vi "prroducer and consumer design patterrn.vi"() -> ()   [LabVIEW 2022 SP3]
uses:
  <vilib>/ptbypt/NI_PtbyPt.lvlib
panel:
  in  "stop":bool
  out "error out":errorcluster
  in  "error in (no error)":errorcluster
  in  "fill":bool
  out "Tank":dbl(slide) scale=0.0..10.0
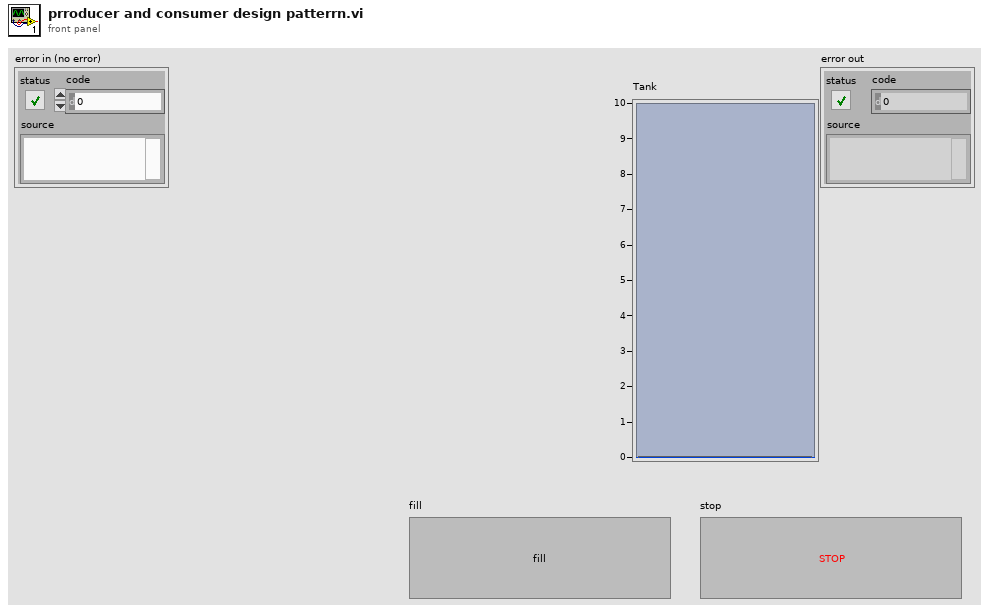
[diagram p1: front panel]
types:
  T1 = enum16{"initialize", "fill", "stop", "button", "errorr"}
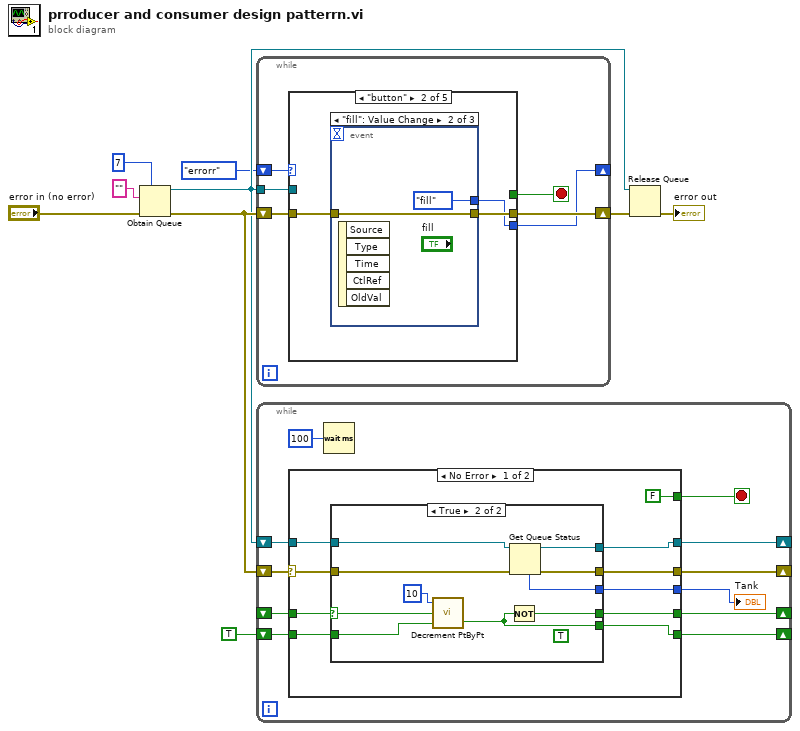
[diagram p0: block diagram]
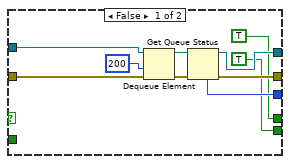
[diagram p2: hidden frame]
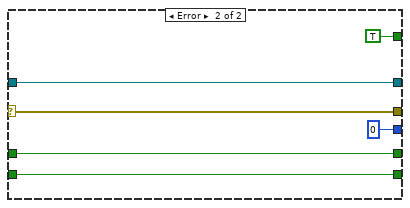
[diagram p3: hidden frame]
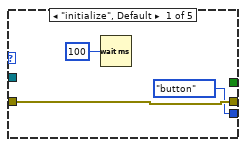
[diagram p4: hidden frame]
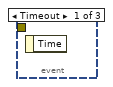
[diagram p5: hidden frame]
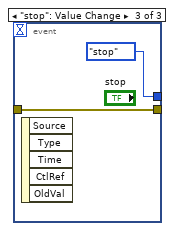
[diagram p6: hidden frame]
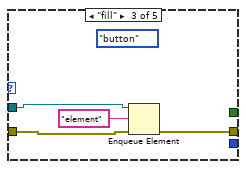
[diagram p7: hidden frame]
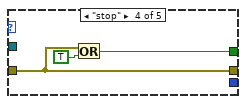
[diagram p8: hidden frame]
diagram:
  n1 = Obtain Queue(max queue size (-1, unlimited)=7, element data type="" ("name (unnamed)"), error in (no error)="error in (no error)") -> (queue out=w4:refnum<queue>, error out=w8:errorcluster)  [unwired: 2 in, 1 out]
  n2 = while {
    tunnel: w4 -> [w14]
    shift-right: [w13] -> w6
    shift-left: w8 -> [w15]
    shift-right: [w11] -> _
    shift-left: T1."errorr" -> [w12]
    stop <- w10 stop-if-true
    n3 = case shown="\"button\"" w12 {
      tunnel: w15 -> [w17 w20 w27 w30 w33]
      tunnel: w14 -> [_ _ w28 _ _]
      tunnel: [w17 w21 w26 w30 w33] -> w13
      tunnel: [T1."button" w19 _ _ _] -> w11
      tunnel: [_ _ _ w32 _] -> w10
      frame "initialize", Default {
        n4 = Wait (ms)(milliseconds to wait=u32 100) -> ()  [unwired: 1 out]
      }
      frame "button" {
        n5 = event shown="[1] \"fill\": Value Change" {
          selector: _ -> [_ _ _]
          dyn-events: _ -> [_ _ _]
          timeout: _ -> [_ _ _]
          tunnel: [_ w23 w24] -> w21
          tunnel: w20 -> [_ w23 w24]
          tunnel: [_ T1."fill" T1."stop"] -> w19
          event Timeout {
            n6 = event-data() -> ()  [unwired: 1 in, 1 out]
          }
          event "fill": Value Change {
            n7 = event-data() -> ()  [unwired: 1 in, 5 out]
          }
          event "stop": Value Change {
            n8 = event-data() -> ()  [unwired: 1 in, 5 out]
          }
        }
      }
      frame "fill" {
        (unwired) T1."button"
        n9 = Enqueue Element(queue=w28, element="element", error in (no error)=w27) -> (error out=w26:errorcluster)  [unwired: 1 in, 2 out]
      }
      frame "stop" {
        n10 = Or(x=w30, y=TRUE) -> (x .or. y?=w32:bool)
      }
      frame "errorr" {
      }
    }
  }
  n11 = while {
    shift-right: [w41] -> _
    shift-left: w4 -> [w44]
    shift-right: [w42] -> _
    shift-left: w8 -> [w43]
    shift-right: [w39] -> _
    shift-left: _ -> [w37]
    shift-right: [w38] -> _
    shift-left: TRUE ("zero crossing") -> [w36]
    stop <- w35 stop-if-true
    n12 = case shown="No Error" w43 {
      selector: w43 -> [w53 w80]
      tunnel: w44 -> [w54 w75]
      tunnel: [w52 w80] -> w42
      tunnel: [w51 w75] -> w41
      tunnel: [w50 0 ("# elements in queue")] -> w40
      tunnel: [w49 w79] -> w39
      tunnel: [w48 w78] -> w38
      tunnel: w37 -> [w47 w79]
      tunnel: w36 -> [w46 w78]
      tunnel: [FALSE TRUE] -> w35
      frame No Error {
        n13 = case shown="True" w47 {
          selector: w47 -> [_ w66]
          tunnel: w54 -> [w64 w74]
          tunnel: w53 -> [w63 w73]
          tunnel: [w59 w72] -> w52
          tunnel: [w60 w71] -> w51
          tunnel: [w58 w70] -> w50
          tunnel: [TRUE w68] -> w49
          tunnel: [TRUE ("zero crossing") w67] -> w48
          tunnel: w46 -> [_ w65]
          frame False {
            n14 = Dequeue Element(queue=w64, timeout in ms (-1)=200, error in (no error)=w63) -> (queue out=w62:refnum<queue>, error out=w61:errorcluster)  [unwired: 2 out]
            n15 = Get Queue Status(queue=w62, error in (no error)=w61) -> (queue out=w60:refnum<queue>, error out=w59:errorcluster, # elements in queue=w58:i32)  [unwired: 1 in, 5 out]
          }
          frame True {
            (unwired) TRUE
            n16 = call <vilib>:"Decrement PtByPt.vi"("initialize"=w65, "activate"=w66, "start"=u32 10) -> ("zero crossing"=w67:bool)  [unwired: 1 out]
            n17 = Not(x=w67) -> (.not. x?=w68:bool)
            n18 = Get Queue Status(queue=w74, error in (no error)=w73) -> (queue out=w71:refnum<queue>, error out=w72:errorcluster, # elements in queue=w70:i32)  [unwired: 1 in, 5 out]
          }
        }
      }
      frame Error {
      }
    }
    "Tank" <- w40
    n19 = Wait (ms)(milliseconds to wait=u32 100) -> ()  [unwired: 1 out]
  }
  n20 = Release Queue(queue=w4, error in (no error)=w6) -> (error out=→"error out":errorcluster)  [unwired: 1 in, 2 out]
